vi "get_first_two_queue_elements.vi"(11 "Waypoint queue":refnum<queue>) -> (1 "Second element":refnum<class "Waypoint.lvclass">, 2 "First element":refnum<class "Waypoint.lvclass">, 3 "Waypoint queue out":refnum<queue>)   [LabVIEW 2013]
doc: "Returns the first two elements off of a waypoint queue. This is so that path planning can get the boat to the next waypoint (1st element) and generally point the boat towards the next waypoint (2nd element).\n\nQueue is unchanged.\n\nEric Schneider, September 2014"
uses:
  Classes/Waypoint/Waypoint.lvclass
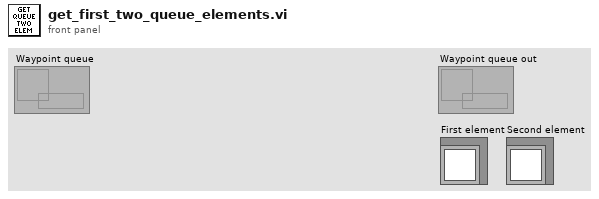
[diagram p1: front panel]
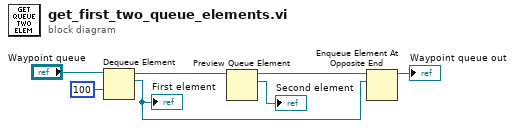
[diagram p0: block diagram]
diagram:
  n1 = Dequeue Element(queue="Waypoint queue", timeout in ms (-1)=100) -> (queue out=w5:refnum<queue>, element=w2:refnum<class "Waypoint.lvclass">)  [unwired: 1 in, 2 out]
  "First element" <- w2
  n2 = Preview Queue Element(queue=w5) -> (queue out=w3:refnum<queue>, element=→"Second element":refnum<class "Waypoint.lvclass">)  [unwired: 2 in, 2 out]
  n3 = Enqueue Element At Opposite End(queue=w3, element=w2) -> (queue out=→"Waypoint queue out":refnum<queue>)  [unwired: 2 in, 2 out]
